vi "ADC_Waveform_Scan_v2.vi"(0 "GPIB Address":T3=8, 1 "Trigger mode":T1, 5 "Ch & spans":T2[](array[typedef])=[{"high limit (10V)"=10.0, "low limit (-10V)"=-10.0, "Ch No"=0, "Var name"="", "Use Latest Calib"=FALSE}] {"low limit (-10V)" format="%.3f"; "high limit (10V)" format="%.3f"}, 7 "number of scans\n(1000)":i32=1000, 9 "scan rate (1000 scans/sec)":dbl=1000.0 format="%.2f", 11 "error in (no error)":errorcluster, 12 "Local Client?":bool, 13 "Current Block No":i32) -> (8 "Binary data":i16[][](array[numeric]), 10 "Actual Sampling rate (Hz)":dbl=1000.0 format="%.2f", 15 "error out":errorcluster)   [LabVIEW 2010]
doc: "This VI acquires the specified number of scans at the specified scan rate and returns all the data acquired. You can trigger the acquisition.\nInput Values:\n\n(i16) GPIB Address The GPIB address of the ADC. You must specify address.\n\n([string]) channels: specifies the set of analog input channels.The default input is channel 0.\n\n(i32) number of scans: the number of scans the VI acquires before the acquisition is complete.\n\n(sgl) scan rate: the number of scans per second to acquire.\n\n([cluster]) input limits: an array of clusters, of which each array element specifies the range limits for the channel(s) in the corresponding element of the channels array. If there are fewer elements in this array than the number of channels,panic. Each cluster contains the following parameters: \n\n (sgl) high limit: specifies the maximum scaled data the\n device measures at a particular channel.\n\n (sgl) low limit: specifies the minimum scaled data the\n device measures at a particular channel.\n\n(bool) clear acquisition:\n\n(sgl) time limit in sec: defines the timeout for the read operation. If the value is -1 (default), LabVIEW calculates the time limit based on the number of scans and the scan rate. If you use a trigger to start the acquisition, you need to specify a longer time limit to include the expected delay between the call to AI Start that enables the acquisition and the trigger event that starts the acquisition. If a timeout occurs, the VI returns any partial data that it acquired, and the error code indicates a timeout. The resolution of the timeout clock is about 55 msec.\n\n\n(cluster) error in: a cluster describing any error conditions prior to this VI's execution. The default input of this cluster is no error. If an error has already occurred, this VI does nothing, it just passes the values of taskID in and error in to taskID out and error out. The error in cluster contains the following parameters: \n\n (bool) status: TRUE if an error has occurred.\n If status is TRUE, this VI does nothing.\n\n (i32) code: the error code associated with an error.\n A value of 0 means no error, a negative value is an error,\n and a positive value is a warning.\n\n (string) source: an indication of where an \n error occurred, usually the name of the VI.\n\nOutput Values:\n\n([[sgl]]) scaled data: a two-dimensional array that contains analog input data in scaled data units. The first dimension holds data for a channel. The second dimension selects which channel.\n\n(sgl) actual scan period: the time between scans, the inverse of the actual scan rate the VI used to acquire the data. This may differ slightly from the requested scan rate, depending on the hardware capabilities.\n\n(cluster) error out: a cluster containing error information. If error in indicated an error, error out contains the same error information. Otherwise, it describes the error status of this VI. Use the General Error Handler utility VI to check the error at the end of your diagram. The error out cluster contains the following parameters: \n\n (bool) status: TRUE if an error has occurred.\n\n (i32) code: the error code associated with an error.\n A value of 0 means no error, a negative value is an error,\n and a positive value is a warning.\n\n (string) source: an indication of where an \n error occurred, usually the name of the VI."
uses:
  ADC_GPIB_address.ctl
  Controls/Ch_and_Spans.ctl
  Controls/Trigger_Mode.ctl
  Globals/Meas_global.vi
  Globals/LDA_meas_global_1.vi
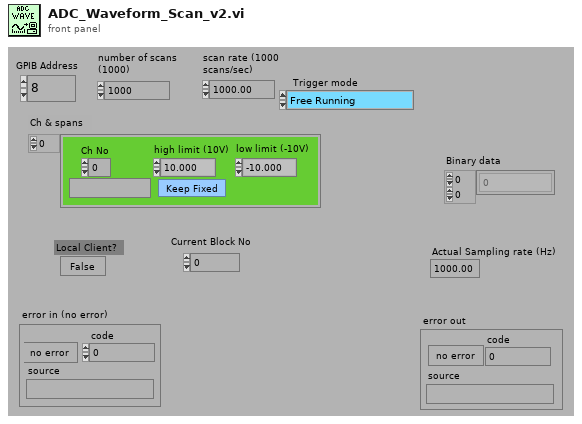
[diagram p1: front panel]
types:
  T1 = typedef "Trigger_Mode.ctl" = enum16{"Free Running", "Start on Trigger", "Trigger Every Block", "Trigger Every Sample"}
  T2 = typedef "Ch_and_Spans.ctl" = cluster{"high limit (10V)":sgl, "low limit (-10V)":sgl, "Ch No":i16, "Var name":string, "Use Latest Calib":bool}
  T3 = typedef "ADC_GPIB_address.ctl" = u8
  T4 = typedef "BSA_info_Cluster.ctl" = cluster{"GPIB Address":string, "No of Check Bytes":i32, "Extra Info":string, "COLOUR":u32, "Wavelength (nm)":dbl}
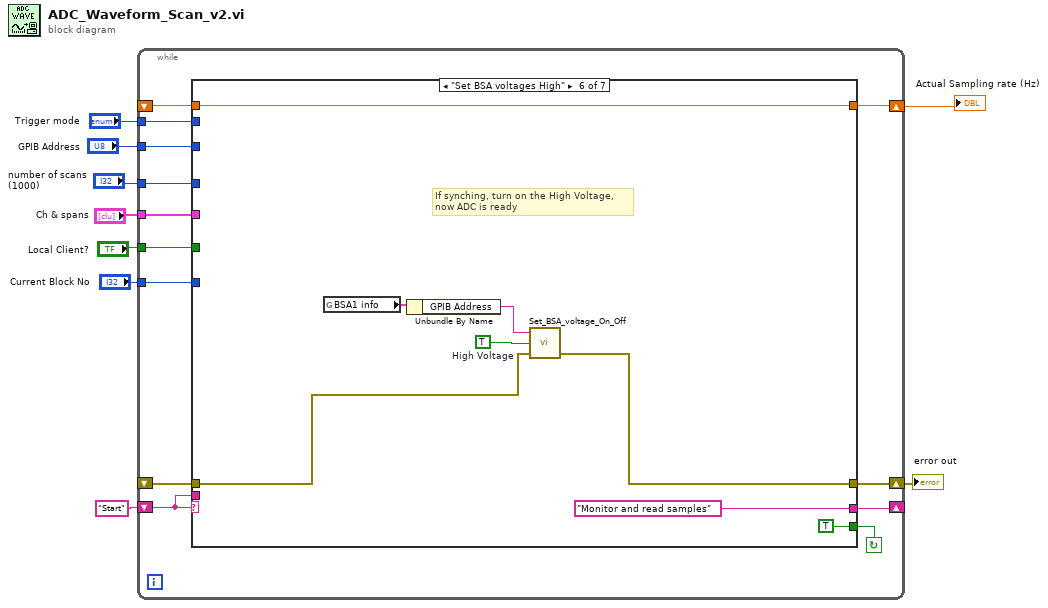
[diagram p0: block diagram]
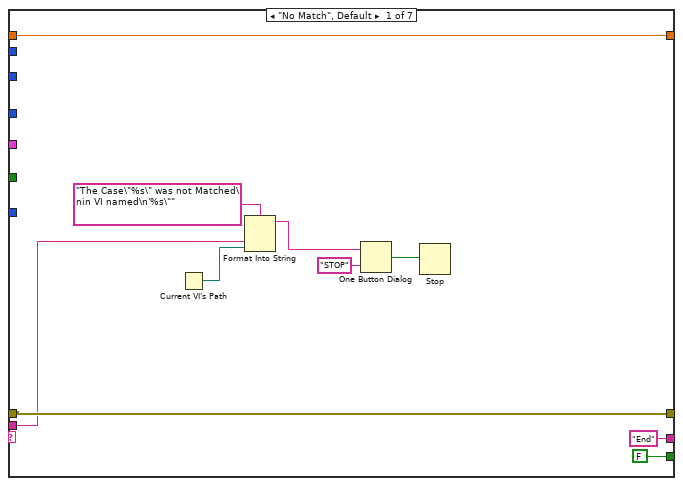
[diagram p2: hidden frame]
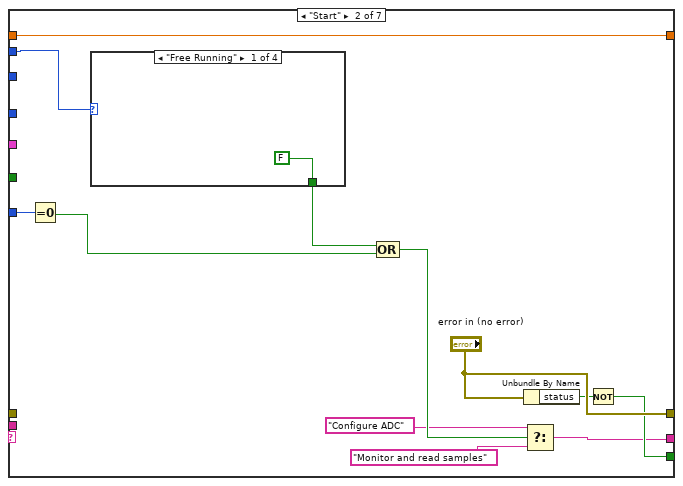
[diagram p3: hidden frame]
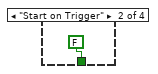
[diagram p4: hidden frame]
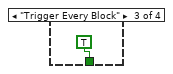
[diagram p5: hidden frame]
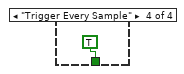
[diagram p6: hidden frame]
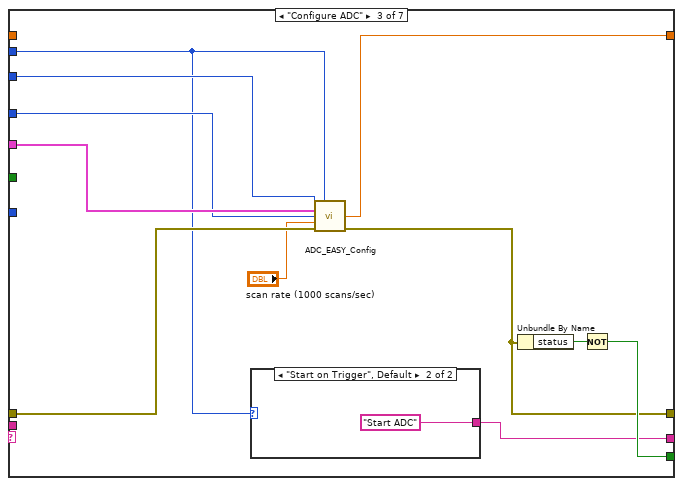
[diagram p7: hidden frame]
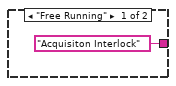
[diagram p8: hidden frame]
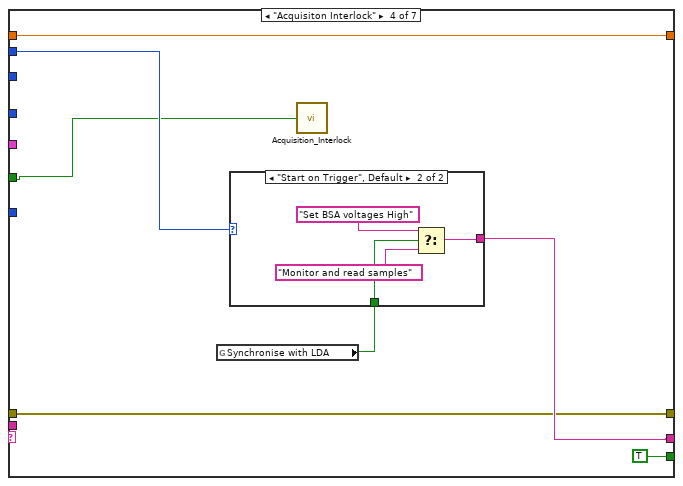
[diagram p9: hidden frame]
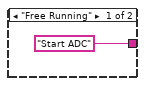
[diagram p10: hidden frame]
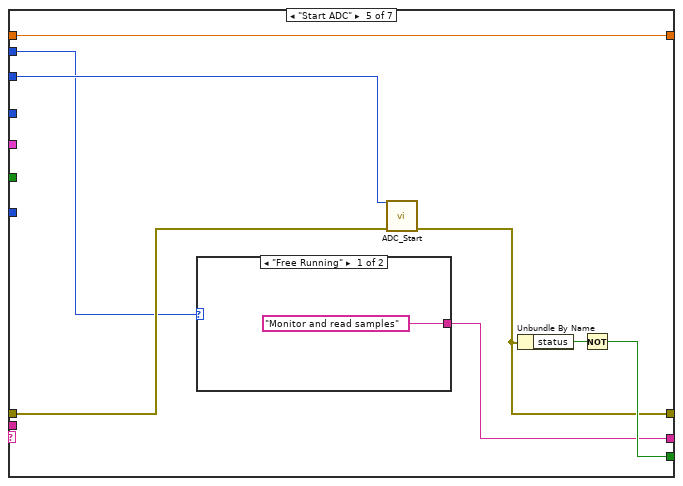
[diagram p11: hidden frame]
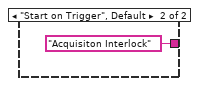
[diagram p12: hidden frame]
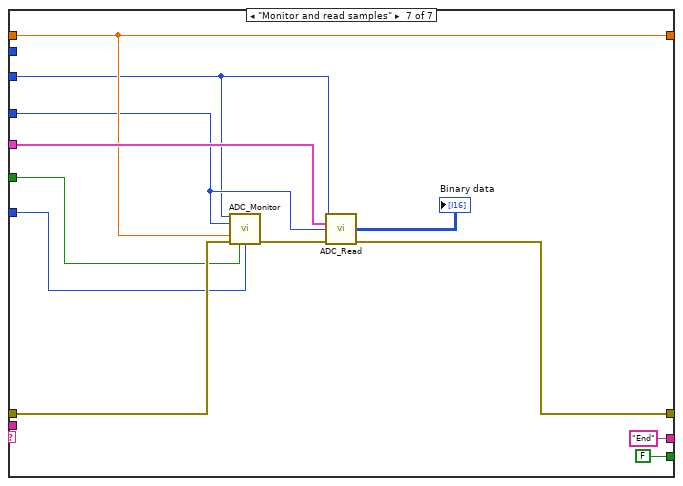
[diagram p13: hidden frame]
diagram:
  n1 = while {
    tunnel: "GPIB Address" -> [w13]
    tunnel: "number of scans\n(1000)" -> [w14]
    shift-left: _ -> [w12]
    shift-right: [w15] -> w2
    tunnel: "Ch & spans" -> [w17]
    tunnel: "Local Client?" -> [w18]
    tunnel: "Current Block No" -> [w19]
    shift-left: _ -> [w16]
    shift-right: [w20] -> w8
    shift-left: "Start" -> [w11]
    shift-right: [w22] -> _
    tunnel: "Trigger mode" -> [w10]
    stop <- w21 continue-if-true
    n2 = case shown="\"Set BSA voltages High\"" w11 {
      tunnel: ["End" ("f") w40 w49 w65 w74 "Monitor and read samples" "End" ("f")] -> w22
      tunnel: [FALSE w42 w56 TRUE w80 TRUE FALSE] -> w21
      tunnel: [w31 "error in (no error)" w51 w64 w78 w85 w100] -> w20
      tunnel: w19 -> [_ w41 _ _ _ _ w94]
      tunnel: w18 -> [_ _ _ w62 _ _ w93]
      tunnel: w17 -> [_ _ w59 _ _ _ w99]
      tunnel: w16 -> [w31 _ w58 w64 w77 w86 w102]
      tunnel: [w32 w39 w55 w68 w76 w90 w98] -> w15
      tunnel: w14 -> [_ _ w53 _ _ _ w96]
      tunnel: w13 -> [_ _ w52 _ w79 _ w95]
      tunnel: w12 -> [w32 w39 _ w68 w76 w90 w98]
      tunnel: w11 -> [w24 _ _ _ _ _ _]
      tunnel: w10 -> [_ w34 w50 w66 w75 _ _]
      frame "No Match", Default {
        n3 = Current VI's Path() -> (path=w25:path)
        n4 = Format Into String(format string="The Case\"%s\" was not Matched\nin VI named\n'%s\"" ("Format String"), w24, w25) -> (resulting string=w28:string)  [unwired: 2 in, 1 out]
        n5 = One Button Dialog(message=w28, button name ("OK")="STOP") -> (true=w26:bool)
        n6 = Stop(stop? (T)=w26) -> ()
      }
      frame "Start" {
        n7 = Equal To 0?(x=w41) -> (x = 0?=w38:bool)
        n8 = case shown="\"Free Running\"" w34 {
          tunnel: [FALSE FALSE TRUE TRUE] -> w33
          frame "Free Running" {
          }
          frame "Start on Trigger" {
          }
          frame "Trigger Every Block" {
          }
          frame "Trigger Every Sample" {
          }
        }
        n9 = Compound Arithmetic op=OR(w33, w38) -> (w37:bool)
        n10 = Unbundle By Name("error in (no error)") -> ("status"=w43:bool)
        n11 = Select(t="Configure ADC", s=w37, f="Monitor and read samples") -> (s? t:f=w40:string)
        n12 = Not(x=w43) -> (.not. x?=w42:bool)
      }
      frame "Configure ADC" {
        n13 = case shown="\"Start on Trigger\", Default" w50 {
          tunnel: ["Acquisiton Interlock" "Start ADC"] -> w49
          frame "Free Running" {
          }
          frame "Start on Trigger", Default {
          }
        }
        n14 = call "ADC_EASY_Config.vi"("GPIB Address"=w52, "Trigger mode"=w50, "Ch & spans"=w59, "buffer size (1000 scans)"=w53, "scan rate (1000 scans/sec)"="scan rate (1000 scans/sec)", "error in (no error)"=w58) -> ("actual scan rate"=w55:dbl, "error out"=w51:errorcluster)  [unwired: 1 in, 7 out]
        n15 = Unbundle By Name(w51) -> ("status"=w57:bool)
        n16 = Not(x=w57) -> (.not. x?=w56:bool)
      }
      frame "Acquisiton Interlock" {
        n17 = global read "Meas_global.vi" "Synchronise with LDA"() -> (w63:bool)
        n18 = case shown="\"Start on Trigger\", Default" w66 {
          tunnel: ["Start ADC" w71] -> w65
          tunnel: w63 -> [_ w73]
          frame "Free Running" {
          }
          frame "Start on Trigger", Default {
            n19 = Select(t="Set BSA voltages High", s=w73, f="Monitor and read samples") -> (s? t:f=w71:string)
          }
        }
        n20 = call "Acquisition_Interlock.vi"("Local Control"=w62) -> ()
      }
      frame "Start ADC" {
        n21 = case shown="\"Free Running\"" w75 {
          tunnel: ["Monitor and read samples" "Acquisiton Interlock"] -> w74
          frame "Free Running" {
          }
          frame "Start on Trigger", Default {
          }
        }
        n22 = call "ADC_Start.vi"("GPIB Address"=w79, "error in (no error)"=w77) -> ("error out"=w78:errorcluster)  [unwired: 5 in, 8 out]
        n23 = Unbundle By Name(w78) -> ("status"=w81:bool)
        n24 = Not(x=w81) -> (.not. x?=w80:bool)
      }
      frame "Set BSA voltages High" {
        w89 = TRUE  # High Voltage
        # "If synching, turn on the High Voltage,\nnow ADC is ready"
        n25 = global read "LDA_meas_global_1.vi" "BSA1 info"() -> (w88:T4)
        n26 = Unbundle By Name(w88) -> ("GPIB Address"=w87:string)
        n27 = call "Set_BSA_voltage_On_Off.vi"("GPIB address"=w87, "High Voltage"=w89, "error in (no error)"=w86) -> ("error out"=w85:errorcluster)  [unwired: 4 out]
      }
      frame "Monitor and read samples" {
        n28 = call "ADC_Monitor.vi"("GPIB Address"=w95, "Chunk Size"=w96, "Sample Rate (Hz)"=w98, "error in (no error)"=w102, "Local Client?"=w93, "Current Block No"=w94) -> ("error out"=w101:errorcluster)  [unwired: 9 out]
        n29 = call "ADC_Read.vi"("GPIB Address"=w95, "Ch & spans"=w99, "number of scans to read"=w96, "error in (no error)"=w101) -> ("binary data"=→"Binary data":i16[][], "error out"=w100:errorcluster)  [unwired: 1 in, 9 out]
      }
    }
  }
  "error out" <- w8
  "Actual Sampling rate (Hz)" <- w2
